vi "Manual Shoot High.vi"(7 "ShootNow":bool, 8 "error in (no error)":errorcluster, 9 "LowSpeed":bool, 10 "MidSpeed":bool, 11 "TopSpeed":bool) -> (0 "error out":errorcluster)   [LabVIEW 2017]
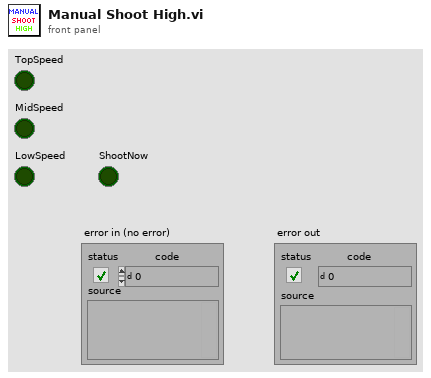
[diagram p1: front panel]
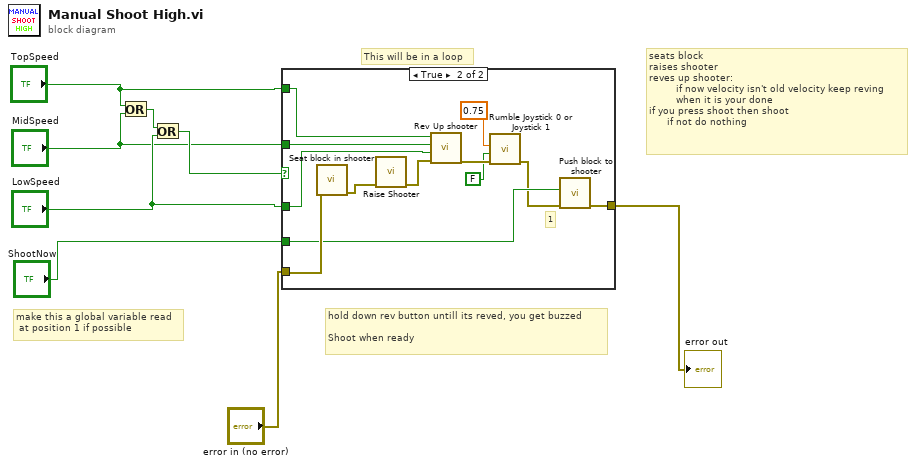
[diagram p0: block diagram]
diagram:
  # "This will be in a loop"
  # "hold down rev button untill its reved, you get buzzed\n\nShoot when ready"
  # "seats block\nraises shooter\nreves up shooter:\n         if now velocity isn't old velocity keep reving\n         when it is your done\nif you press shoot then shoot\n      if not do nothing"
  # "make this a global variable read\n at position 1 if possible"
  n1 = Or(x="TopSpeed", y="MidSpeed") -> (x .or. y?=w6:bool)
  n2 = Or(x=w6, y="LowSpeed") -> (x .or. y?=w5:bool)
  n3 = case shown="True" w5 {
    tunnel: "error in (no error)" -> [w9 w20]
    tunnel: [w9 w18] -> w7
    tunnel: "LowSpeed" -> [_ w15]
    tunnel: "MidSpeed" -> [_ w16]
    tunnel: "TopSpeed" -> [_ w17]
    tunnel: "ShootNow" -> [_ w14]
    frame False {
    }
    frame True {
      # "1"
      n4 = call "Seat block in shooter.vi"("error in (no error)"=w20) -> ("error out"=w19:errorcluster)  [unwired: 10 in]
      n5 = call "Raise Shooter.vi"("error in (no error)"=w19) -> ("error out"=w21:errorcluster)  [unwired: 10 in]
      n6 = call "Rev Up shooter.vi"("error in (no error)"=w21, "LowSpeed"=w15, "MidSpeed"=w16, "TopSpeed"=w17) -> ("error out"=w13:errorcluster)  [unwired: 7 in]
      n7 = call "Rumble Joystick 0 or Joystick 1.vi"("error in (no error)"=w13, "Joystick 0?"=FALSE, "Magnitude of buzz"=0.75) -> ("error out"=w12:errorcluster)  [unwired: 8 in]
      n8 = call "Push block to shooter.vi"("error in (no error)"=w12, "Shoot?"=w14) -> ("error out"=w18:errorcluster)  [unwired: 9 in]
    }
  }
  "error out" <- w7
